vi "Advanced Cut - Draw Time Series.vi"(7 "Parameter Time Series":T1(array[cluster]) caption="X-off    Y-off     Gain   Inv Filt Dot Int                      Channel                                  Vis" {"time offset" format="%.3f"; "Gain" format="%.1f"; "Offset" format="%.1f"; "List 1" items=["-", "Hz Velocity-in-Head", "-", "Hy Velocity-in-Head", "-", "Hx Velocity-in-Head", "Hl Velocity-in-Head", "Hr Velocity-in-Head", "-", "Ly Position-in-Head", "Lz Position-in-Head", "-", "Ly Velocity-in-Head", "Lz Velocity-in-Head", "-", "-", "-", "-", "-", "-", "-", "-", "-", "-"]}, 8 "error in (no error)":errorcluster, 9 "Sample Rate":dbl, 10 "Data":dbl[][](array[numeric]), 11 "Time Series Graph in":refnum<vi>) -> (0 "error out":errorcluster, 3 "Time Series Graph out":refnum<vi>)   [LabVIEW 2016]
uses:
  <vilib>/Analysis/1siggen.llb/Ramp Pattern by Samples.vi
  <vilib>/Analysis/NI_AALBase.lvlib
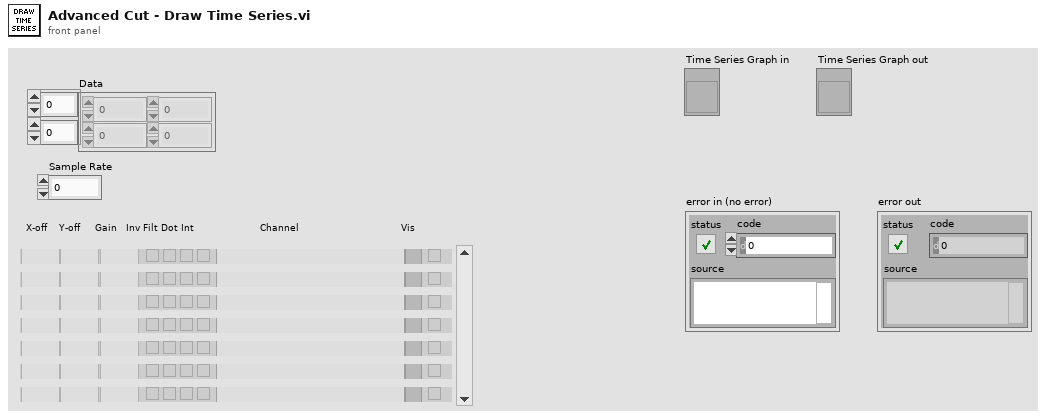
[diagram p1: front panel]
types:
  T1 = cluster{"time offset":dbl, "Offset":dbl, "Gain":dbl, "inverse":bool, "filter data":bool, "dots":bool, "interpolate":bool, "List 1":u16, "Color Box":u32, "Boolean":bool}[]
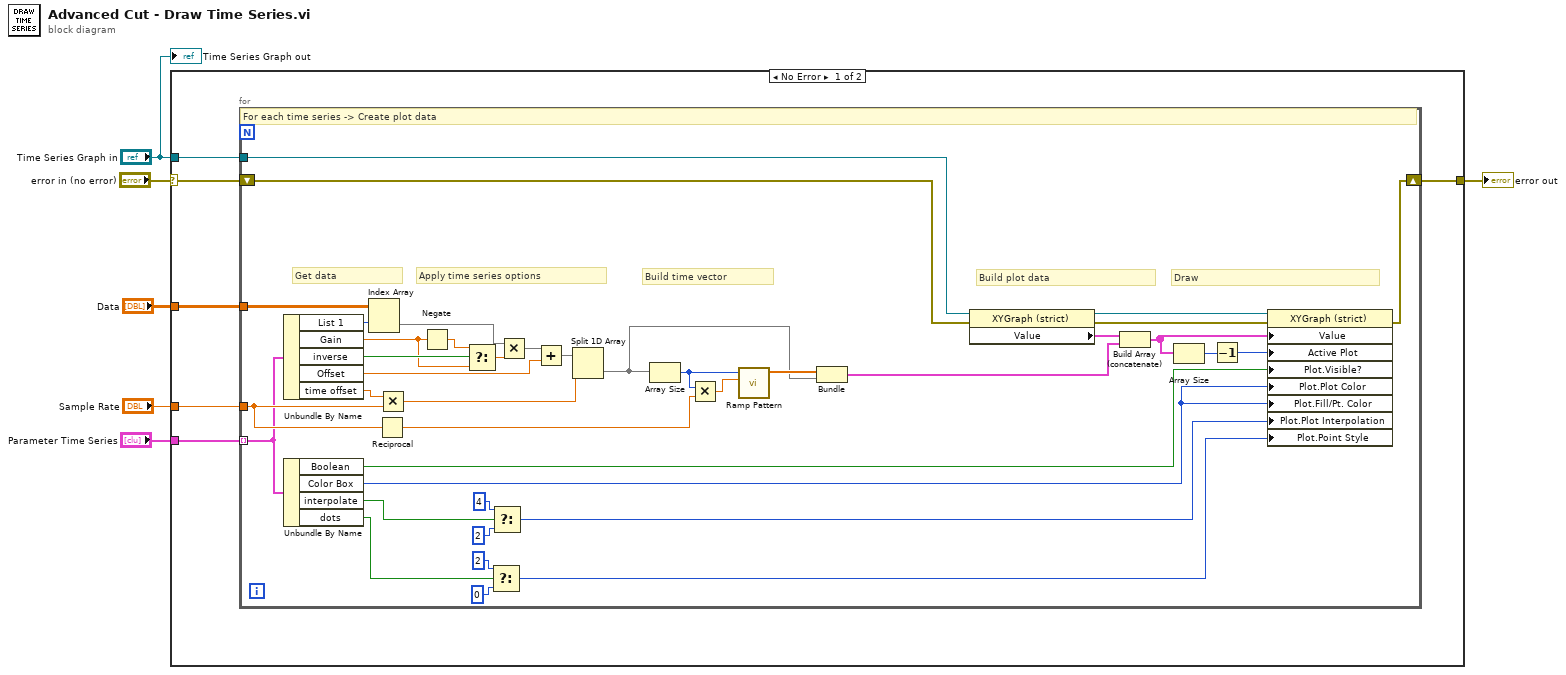
[diagram p0: block diagram]
diagram:
  n1 = case shown="No Error" "error in (no error)" {
    selector: "error in (no error)" -> [w8 w52]
    tunnel: "Time Series Graph in" -> [w12 _]
    tunnel: "Data" -> [w11 _]
    tunnel: "Sample Rate" -> [w10 _]
    tunnel: "Parameter Time Series" -> [w9 _]
    tunnel: [w7 w52] -> w1
    frame No Error {
      n2 = for {
        tunnel: w11 -> [w51]
        tunnel: w10 -> [w39]
        tunnel: w9 -> [w19] mode=indexing
        tunnel: w12 -> [w18]
        shift-right: [w13] -> w7
        shift-left: w8 -> [w15]
        # "Draw"
        # "Build plot data"
        # "Build time vector"
        # "Apply time series options"
        # "Get data"
        # "For each time series -> Create plot data"
        n3 = Unbundle By Name(w19) -> ("List 1"=w50:u16, "Gain"=w47:dbl, "inverse"=w49:bool, "Offset"=w43:dbl, "time offset"=w42:dbl)
        n4 = Unbundle By Name(w19) -> ("Boolean"=w29:bool, "Color Box"=w24:u32, "interpolate"=w28:bool, "dots"=w21:bool)
        n5 = Index Array(array=w51, index (row)=w50) -> (element=w45:dbl[])  [unwired: 1 in]
        n6 = Reciprocal(x=w39) -> (1/x=w37:dbl)
        n7 = Multiply(x=w42, y=w39) -> (x*y=w41:dbl)
        n8 = Negate(x=w47) -> (-x=w48:dbl)
        n9 = Select(t=w48, s=w49, f=w47) -> (s? t:f=w46:dbl)
        n10 = Select(t=u8 2 ("Plot.Point Style"), s=w21, f=u8 0 ("Plot.Point Style")) -> (s? t:f=w20:u8)
        n11 = Select(t=u8 4 ("Plot.Point Style"), s=w28, f=u8 2 ("Plot.Point Style")) -> (s? t:f=w25:u8)
        n12 = Multiply(x=w45, y=w46) -> (x*y=w44:dbl[])
        n13 = Add(x=w44, y=w43) -> (x+y=w40:dbl[])
        n14 = Split 1D Array(array=w40, index=w41) -> (second subarray=w34:dbl[])  [unwired: 1 out]
        n15 = Array Size(array=w34) -> (size(s)=w38:i32)
        n16 = Multiply(x=w38, y=w37) -> (x*y=w36:dbl)
        n17 = call-poly <vilib>:"Ramp Pattern.vi"("end"=w36, "samples"=w38) -> ("Ramp Pattern"=w35:dbl[])  [unwired: 8 in, 1 out]
        n18 = Bundle("Ramp Pattern"=w35, w34) -> (w33:cluster{"Ramp Pattern":dbl[], dbl[]})  [unwired: 1 in]
        n19 = property on="Property Node" class="XYGraph (strict)"(reference=w18, error in=w15) -> (reference out=w16:refnum<vi>, error out=w14:errorcluster, "Value"=w17:cluster{"Ramp Pattern":dbl[], dbl[]}[])
        n20 = Build Array (concatenate)(w17, w33) -> (w32:cluster{"Ramp Pattern":dbl[], dbl[]}[])
        n21 = Array Size(array=w32) -> (size(s)=w31:i32)
        n22 = Decrement(x=w31) -> (x-1=w30:i32)
        n23 = property on="Property Node" class="XYGraph (strict)"(reference=w16, error in=w14, "Value"=w32, "Active Plot"=w30, "Plot.Visible?"=w29, "Plot.Plot Color"=w24, "Plot.Fill/Pt. Color"=w24, "Plot.Plot Interpolation"=w25, "Plot.Point Style"=w20) -> (error out=w13:errorcluster)  [unwired: 1 out]
      }
    }
    frame Error {
    }
  }
  "error out" <- w1
  "Time Series Graph out" <- "Time Series Graph in"
